vi "Array of I16_Get Index.vi"(8 "error in (no error)":errorcluster, 9 "Default":i16[](array[numeric]), 11 "Tag Name":string) -> (0 "error out":errorcluster, 3 "Index":i32)   [LabVIEW 2016, in "CVT.lvlib" / "Current Value Table.lvlib"]
doc: "This VI retrieves the memory index of a single value as an I32. Since this value is an I32 and has no data associated with it, you must make sure that you use the index read and write for the appropriate type. This VI will check to make sure that the tag name specified matches with the data type specified."
uses:
  <vilib>/NI/Current Value Table/Current Value Table.lvlib
  <vilib>/NI/Current Value Table/FGVs/Tag Memory Methods.ctl
  <vilib>/NI/Current Value Table/DataTypes/Array of I16_Type To Enum.vi
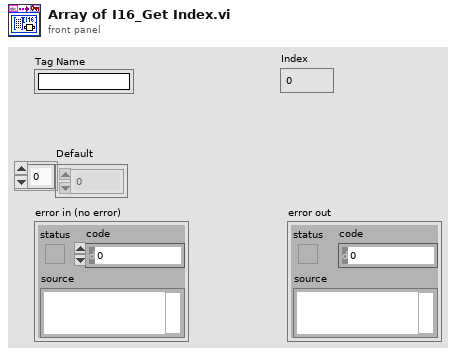
[diagram p1: front panel]
types:
  T1 = typedef "CVT.lvlib/Current Value Table.lvlib/Tag Memory Methods.ctl" = enum16{"Clear", "Read Tag Index", "Read Tag Indices", "Generate Group", "Add Tag", "Overwrite Tag", "Read Description", "Get Stored Tags"}
  T2 = typedef "CVT.lvlib/Current Value Table.lvlib/Data Types.ctl" = enum16{"Double", "Single", "I64", "I32", "I16", "I8", "U64", "U32", "U16", "U8", "String", "Boolean", "Array of U8", "Array of U16", "Array of U32", "Array of U64", "Array of I64", "Array of I32", "Array of I16", "Array of I8", "Array of Double", "Array of Single", "Array of Boolean", "Array of String"}
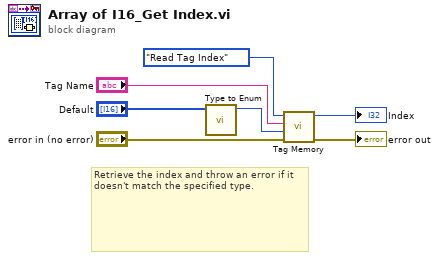
[diagram p0: block diagram]
diagram:
  # "Retrieve the index and throw an error if it doesn't match the specified type."
  n1 = call-poly <vilib>:"Type to Enum.vi"("Default"="Default") -> ("Data Type Enum"=w7:T2)  [unwired: 10 in]
  n2 = call <vilib>:"Tag Memory.vi"("error in (no error)"="error in (no error)", "Expected Type"=w7, "Tag"="Tag Name", "Method"=Tag_Memory_Methods."Read Tag Index") -> ("error out"=→"error out":errorcluster, "Index Out"=→"Index":i32)  [unwired: 2 in, 4 out]
